vi "encrypt DAT to UFS v1_1.vi"() -> ()   [LabVIEW 2020]
uses:
  <vilib>/Utility/file.llb/Read Delimited Spreadsheet (DBL).vi
panel:
  in  "add spectra":bool
  in  "N":i32
  out "all t":dbl[](array[numeric])
  out "all w":dbl[](array[numeric])
  out "X size":i32
  out "Y size":i32
  in  "colors":u32[](array[colorbox])=[153, 16776960, 16711680]
  in  "Save":bool
  in  "Load":bool
  in  "stop":bool
  out "selected path":path
  out "Loaded data":dbl[][](graph)
  # "Add first spectrum N times at the beginning\n(for chirp correction, undo is not available)"
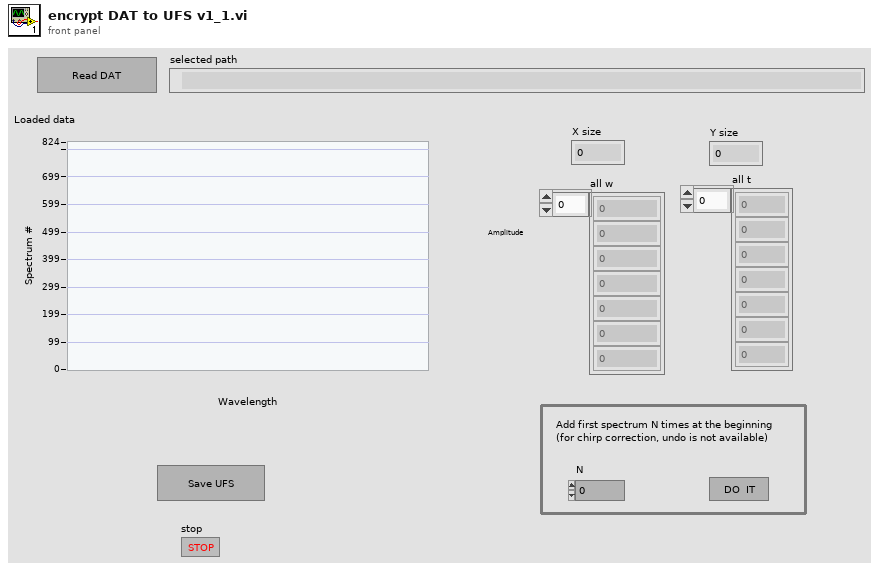
[diagram p1: front panel]
types:
  T1 = enum16{"big-endian, network order", "native, host order", "little-endian"}
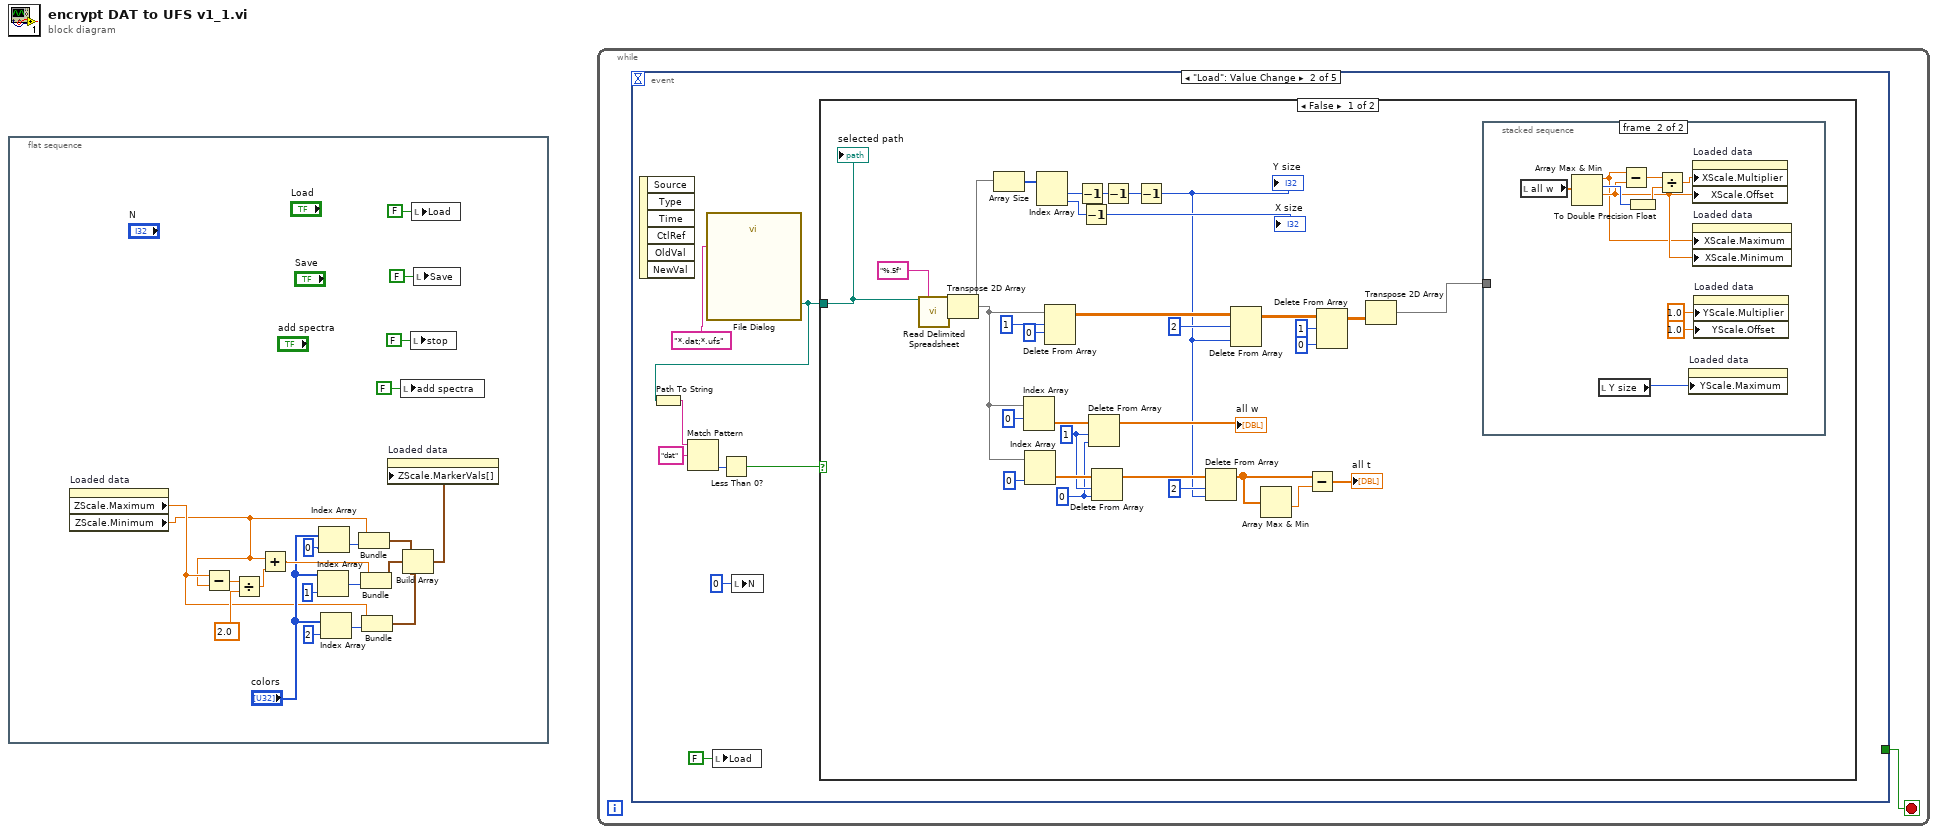
[diagram p0: block diagram]
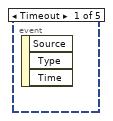
[diagram p2: hidden frame]
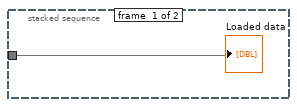
[diagram p3: hidden frame]
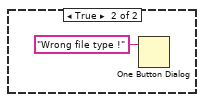
[diagram p4: hidden frame]
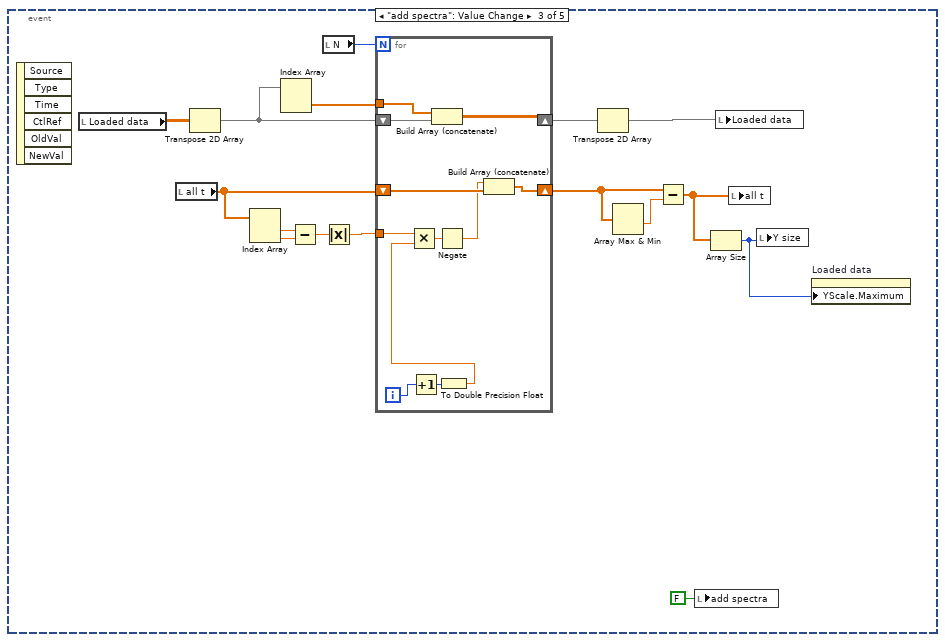
[diagram p5: hidden frame]
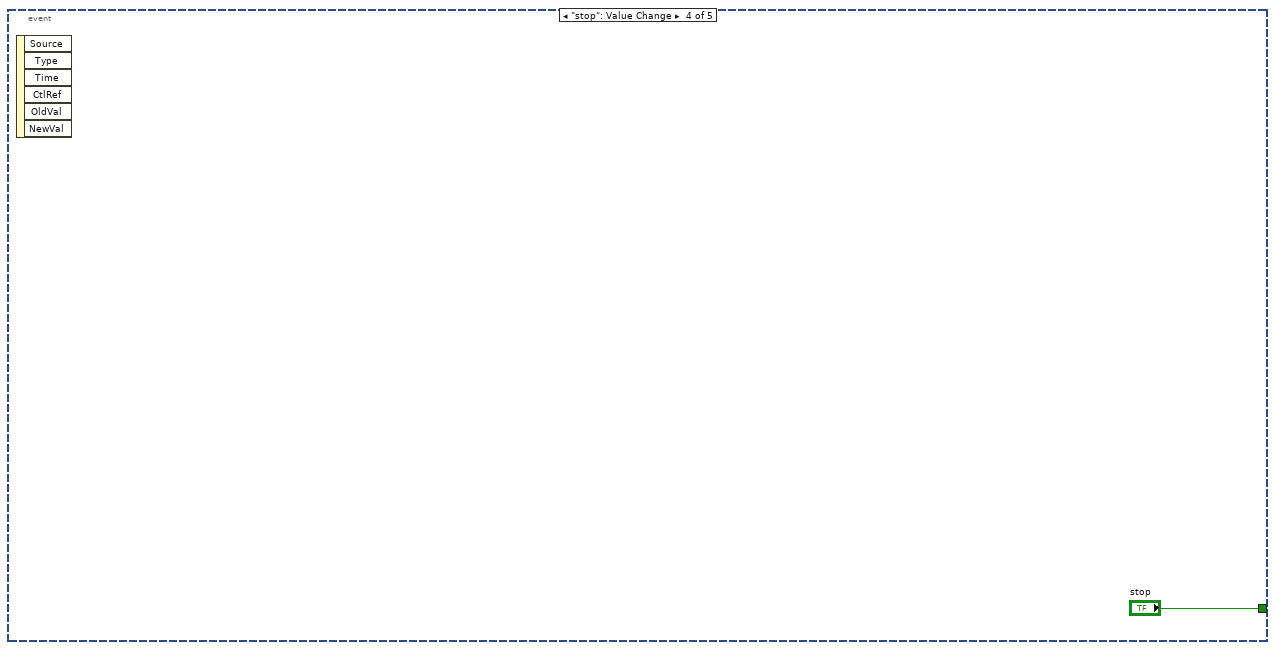
[diagram p6: hidden frame]
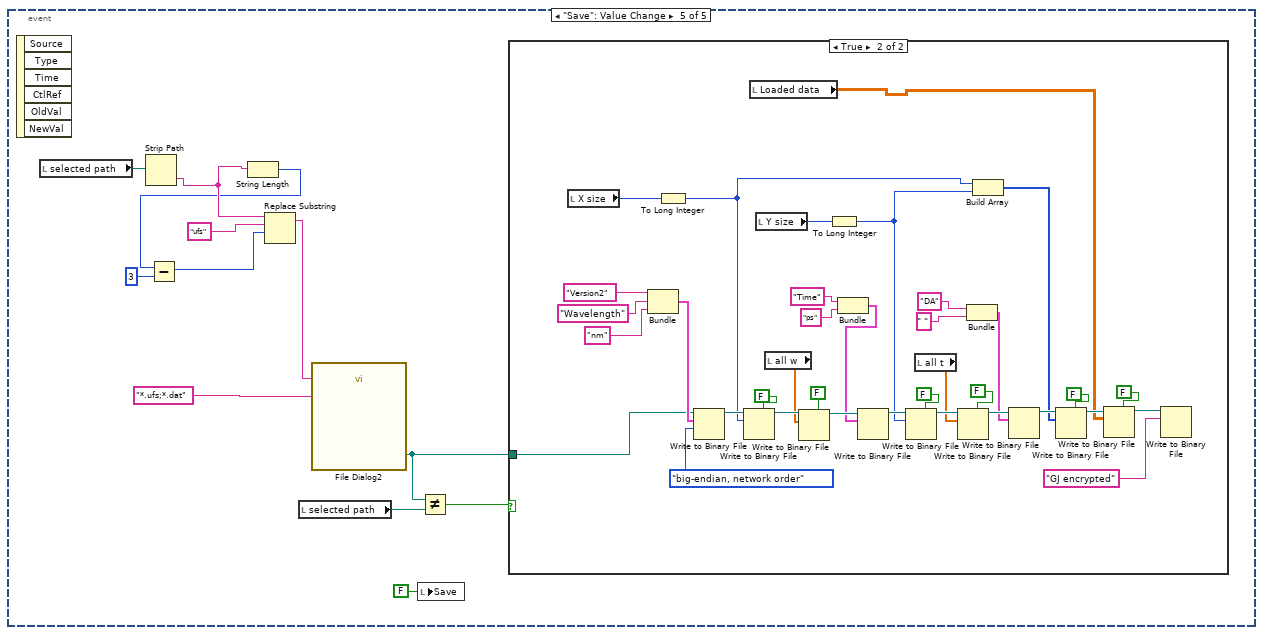
[diagram p7: hidden frame]
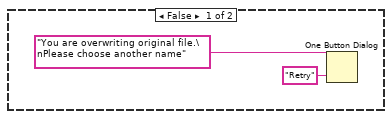
[diagram p8: hidden frame]
diagram:
  n1 = flat-sequence {
    frame #0 {
      n2 = property on="Loaded data" class="IntGraph (strict)"() -> ("ZScale.Maximum"=w4:dbl, "ZScale.Minimum"=w3:dbl)  [unwired: 2 in, 2 out]
      n3 = Subtract(x=w4, y=w3) -> (x-y=w15:dbl)
      n4 = Divide(x=w15, y=2.0) -> (x/y=w17:dbl)
      n5 = Add(x=w3, y=w17) -> (x+y=w18:dbl)
      n6 = Index Array(array="colors", index=1) -> (element=w10:u32)
      n7 = Index Array(array="colors", index=0) -> (element=w11:u32)
      n8 = Index Array(array="colors", index=2) -> (element=w9:u32)
      n9 = Bundle("ZScale.Minimum"=w3, w11) -> (w8:cluster{"ZScale.Minimum":dbl, u32})  [unwired: 1 in]
      n10 = Bundle(w18, w10) -> (w7:cluster{dbl, u32})  [unwired: 1 in]
      n11 = Bundle("ZScale.Maximum"=w4, w9) -> (w6:cluster{"ZScale.Maximum":dbl, u32})  [unwired: 1 in]
      n12 = local write "add spectra"(FALSE ("add spectra")) -> ()
      n13 = Build Array(w8, w7, w6) -> (w2:cluster{"ZScale.Maximum":dbl, u32}[])
      n14 = property on="Loaded data" class="IntGraph (strict)"("ZScale.MarkerVals[]"=w2) -> ()  [unwired: 2 in, 2 out]
      n15 = local write "stop"(FALSE ("stop")) -> ()
      n16 = local write "Load"(FALSE ("Load")) -> ()
      n17 = local write "Save"(FALSE ("Save")) -> ()
    }
  }
  n18 = while {
    stop <- w22 stop-if-true
    n19 = event shown="[1] \"Load\": Value Change" {
      selector: _ -> [_ _ _ _ _]
      dyn-events: _ -> [_ _ _ _ _]
      timeout: _ -> [_ _ _ _ _]
      tunnel: [_ _ _ "stop" _] -> w22
      event Timeout {
        n20 = event-data() -> ()  [unwired: 1 in, 3 out]
      }
      event "Load": Value Change {
        n21 = event-data() -> ()  [unwired: 1 in, 6 out]
        n22 = call "File Dialog"("pattern (all files)"="*.dat;*.ufs") -> ("selected path"=w28:path)  [unwired: 11 in, 3 out]
        n23 = Path To String(path=w28) -> (string=w26:string)
        n24 = Match Pattern(string=w26, regular expression="dat") -> (offset past match=w25:i32)  [unwired: 1 in, 3 out]
        n25 = local write "Load"(FALSE ("Load")) -> ()
        n26 = Less Than 0?(x=w25) -> (x < 0?=w24:bool)
        n27 = local write "N"(0 ("N")) -> ()
        n28 = case shown="False" w24 {
          tunnel: w28 -> [w62 _]
          frame False {
            w51 = 0 ("index")
            w52 = 1 ("length")
            n29 = call-poly <vilib>:"Read Delimited Spreadsheet.vi"("file path (dialog if empty)"=w62, "format (%.3f)"="%.5f") -> ("all rows"=w46:dbl[][])  [unwired: 8 in, 5 out]
            n30 = Transpose 2D Array(2D array=w46) -> (transposed array=w31:dbl[][])
            n31 = Array Size(array=w31) -> (size(s)=w60:i32[])
            n32 = Index Array(array=w31, index (row)=0) -> (element=w58:dbl[])  [unwired: 1 in]
            n33 = Index Array(array=w31, index (col)=0 ("disabled index (col)")) -> (element=w55:dbl[])  [unwired: 1 in]
            n34 = Index Array(array=w60) -> (element #1=w40:i32, element #2=w59:i32)  [unwired: 2 in]
            n35 = Delete From Array(array=w31, length=1, index (row)=0) -> (array with subset deleted=w45:dbl[][])  [unwired: 1 in, 1 out]
            n36 = Decrement(x=w40) -> (x-1=w39:i32)
            n37 = Decrement(x=w59) -> (x-1=→"X size":i32)
            n38 = Delete From Array(array=w58, length=w52, index=w51) -> (array with subset deleted=→"all w":dbl[])  [unwired: 1 out]
            n39 = Delete From Array(array=w55, length=w52, index=w51) -> (array with subset deleted=w49:dbl[])  [unwired: 1 out]
            n40 = Decrement(x=w39) -> (x-1=w33:i32)
            n41 = Decrement(x=w33) -> (x-1=w32:i32)
            "Y size" <- w32
            n42 = Delete From Array(array=w49, length=2, index=w32) -> (array with subset deleted=w35:dbl[])  [unwired: 1 out]
            n43 = Delete From Array(array=w45, length=2, index (row)=w32) -> (array with subset deleted=w42:dbl[][])  [unwired: 1 in, 1 out]
            n44 = Array Max & Min(array=w35) -> (min value=w50:dbl)  [unwired: 3 out]
            n45 = Subtract(x=w35, y=w50) -> (x-y=→"all t":dbl[])
            n46 = Delete From Array(array=w42, length=1, index (col)=0 ("disabled index (col)")) -> (array with subset deleted=w38:dbl[][])  [unwired: 1 in, 1 out]
            n47 = Transpose 2D Array(2D array=w38) -> (transposed array=w47:dbl[][])
            n48 = stacked-sequence {
              tunnel: w47 -> [w63 _]
              frame #0 {
                "Loaded data" <- w63
              }
              frame #1 {
                n49 = local read "all w"() -> (w69:dbl[])
                n50 = Array Max & Min(array=w69) -> (max value=w67:dbl, max index (indices)=w73:i32, min value=w68:dbl)  [unwired: 1 out]
                n51 = local read "Y size"() -> (w64:i32)
                n52 = Subtract(x=w67, y=w68) -> (x-y=w70:dbl)
                n53 = To Double Precision Float(number=w73) -> (double precision float=w72:dbl)
                n54 = Divide(x=w70, y=w72) -> (x/y=w71:dbl)
                n55 = property on="Loaded data" class="IntGraph (strict)"("YScale.Maximum"=w64) -> ()  [unwired: 2 in, 2 out]
                n56 = property on="Loaded data" class="IntGraph (strict)"("XScale.Multiplier"=w71, "XScale.Offset"=w68) -> ()  [unwired: 2 in, 2 out]
                n57 = property on="Loaded data" class="IntGraph (strict)"("XScale.Maximum"=w67, "XScale.Minimum"=w68) -> ()  [unwired: 2 in, 2 out]
                n58 = property on="Loaded data" class="IntGraph (strict)"("YScale.Multiplier"=1.0 ("Y Scale.Offset and Multiplier:Multiplier"), "YScale.Offset"=1.0 ("Y Scale.Offset and Multiplier:Offset")) -> ()  [unwired: 2 in, 2 out]
              }
            }
            "selected path" <- w62
          }
          frame True {
            n59 = One Button Dialog(message="Wrong file type !") -> ()  [unwired: 1 in, 1 out]
          }
        }
      }
      event "add spectra": Value Change {
        n60 = event-data() -> ()  [unwired: 1 in, 6 out]
        n61 = local read "Loaded data"() -> (w85:dbl[][])
        n62 = local read "all t"() -> (w83:dbl[])
        n63 = Transpose 2D Array(2D array=w85) -> (transposed array=w77:dbl[][])
        n64 = Index Array(array=w83) -> (element #1=w88:dbl, element #2=w89:dbl)  [unwired: 2 in]
        n65 = Index Array(array=w77) -> (element=w84:dbl[])  [unwired: 2 in]
        n66 = Subtract(x=w88, y=w89) -> (x-y=w87:dbl)
        n67 = local read "N"() -> (w86:i32)
        n68 = Absolute Value(x=w87) -> (abs(x)=w82:dbl)
        n69 = for {
          N: w86 -> [_]
          shift-right: [w99] -> w78
          shift-left: w77 -> [w100]
          tunnel: w84 -> [w101]
          tunnel: w82 -> [w97]
          shift-right: [w91] -> w81
          shift-left: w83 -> [w98]
          i -> [w96]
          n70 = Increment(x=w96) -> (x+1=w95:i32)
          n71 = Build Array (concatenate)(w101, w100) -> (w99:dbl[][])
          n72 = To Double Precision Float(number=w95) -> (double precision float=w94:dbl)
          n73 = Multiply(x=w97, y=w94) -> (x*y=w93:dbl)
          n74 = Negate(x=w93) -> (-x=w92:dbl)
          n75 = Build Array (concatenate)(w92, w98) -> (w91:dbl[])
        }
        n76 = Transpose 2D Array(2D array=w78) -> (transposed array=w76:dbl[][])
        n77 = Array Max & Min(array=w81) -> (min value=w80:dbl)  [unwired: 3 out]
        n78 = Subtract(x=w81, y=w80) -> (x-y=w79:dbl[])
        n79 = local write "add spectra"(FALSE ("add spectra")) -> ()
        n80 = Array Size(array=w79) -> (size(s)=w75:i32)
        n81 = local write "Loaded data"(w76) -> ()
        n82 = local write "all t"(w79) -> ()
        n83 = local write "Y size"(w75) -> ()
        n84 = property on="Loaded data" class="IntGraph (strict)"("YScale.Maximum"=w75) -> ()  [unwired: 2 in, 2 out]
      }
      event "stop": Value Change {
        n85 = event-data() -> ()  [unwired: 1 in, 6 out]
      }
      event "Save": Value Change {
        n86 = event-data() -> ()  [unwired: 1 in, 6 out]
        n87 = local read "selected path"() -> (w112:path)
        n88 = Strip Path(path=w112) -> (name=w111:string)  [unwired: 1 out]
        n89 = String Length(string=w111) -> (length=w110:i32)
        n90 = Subtract(x=w110, y=3) -> (x-y=w109:i32)
        n91 = Replace Substring(3:w109, 4:"ufs" ("substring (\"\")"), 5:w111) -> (1:w106:string)  [unwired: 1 in, 1 out]
        n92 = local read "selected path"() -> (w104:path)
        n93 = call "File Dialog2"("default name"=w106, "pattern (all files)"="*.ufs;*.dat" ("pattern label")) -> ("selected path"=w105:path)  [unwired: 10 in, 3 out]
        n94 = local write "Save"(FALSE ("Save")) -> ()
        n95 = Not Equal?(x=w105, y=w104) -> (x != y?=w103:bool)
        n96 = case shown="True" w103 {
          tunnel: w105 -> [_ w117]
          frame False {
            n97 = One Button Dialog(message="You are overwriting original file.\nPlease choose another name", button name ("OK")="Retry") -> ()  [unwired: 1 out]
          }
          frame True {
            n98 = local read "X size"() -> (w127:i32)
            n99 = Bundle("Version2", "Wavelength", "nm") -> (w143:cluster{string, string, string})  [unwired: 1 in]
            n100 = To Long Integer(number=w127) -> (32bit integer=w123:i32)
            n101 = Write to Binary File(file (use dialog)=w117, data=w143, 9:T1."big-endian, network order" ("byte order (0:big-endian, network order)")) -> (refnum out=w144:refnum<file>)  [unwired: 3 in, 2 out]
            n102 = Write to Binary File(file (use dialog)=w144, data=w123, 5:FALSE ("prepend array or string size? (T)")) -> (refnum out=w145:refnum<file>)  [unwired: 3 in, 2 out]
            n103 = local read "Loaded data"() -> (w120:dbl[][])
            n104 = local read "Y size"() -> (w126:i32)
            n105 = local read "all w"() -> (w134:dbl[])
            n106 = Write to Binary File(file (use dialog)=w145, data=w134, 5:FALSE ("prepend array or string size? (T)")) -> (refnum out=w146:refnum<file>)  [unwired: 3 in, 2 out]
            n107 = To Long Integer(number=w126) -> (32bit integer=w122:i32)
            n108 = Bundle("Time", "ps") -> (w131:cluster{string, string})  [unwired: 1 in]
            n109 = Write to Binary File(file (use dialog)=w146, data=w131) -> (refnum out=w147:refnum<file>)  [unwired: 4 in, 2 out]
            n110 = Write to Binary File(file (use dialog)=w147, data=w122, 5:FALSE ("prepend array or string size? (T)")) -> (refnum out=w148:refnum<file>)  [unwired: 3 in, 2 out]
            n111 = local read "all t"() -> (w133:dbl[])
            n112 = Write to Binary File(file (use dialog)=w148, data=w133, 5:FALSE ("prepend array or string size? (T)")) -> (refnum out=w149:refnum<file>)  [unwired: 3 in, 2 out]
            n113 = Bundle("DA", " ") -> (w128:cluster{string, string})  [unwired: 1 in]
            n114 = Build Array(w123, w122) -> (w125:i32[])
            n115 = Write to Binary File(file (use dialog)=w149, data=w128) -> (refnum out=w150:refnum<file>)  [unwired: 4 in, 2 out]
            n116 = Write to Binary File(file (use dialog)=w150, data=w125, 5:FALSE ("prepend array or string size? (T)")) -> (refnum out=w151:refnum<file>)  [unwired: 3 in, 2 out]
            n117 = Write to Binary File(file (use dialog)=w151, data=w120, 5:FALSE ("prepend array or string size? (T)")) -> (refnum out=w152:refnum<file>)  [unwired: 3 in, 2 out]
            n118 = Write to Binary File(file (use dialog)=w152, data="GJ encrypted") -> ()  [unwired: 4 in, 3 out]
          }
        }
      }
    }
  }
